vi "UDP Data Link - Driver Utilities - Launch Asynch UDP Loop.vi"(4 "In4Ver":u16, 5 "Rx Initial Values":dbl[](array[numeric]), 6 "SourceNodeName":string, 7 "Status Notifier":refnum<notifier>, 8 "error in (no error)":errorcluster, 9 "Rx Data FIFO":refnum<k33>, 10 "Tx Data FIFO":refnum<k33>, 11 "Device Reference in":T1 format="%.0x") -> (0 "error out":errorcluster)   [LabVIEW 2012, in "UDP Data Link Engine.lvlib"]
doc: "This VI launches the Asynchronous UDP Loop VI in a parallel data space. Before running the asynch VI, it initializes the input data on that VI with the Rx and Tx Data FIFO references, SourceNodeName, In4Ver, UDP Port, IP of Local NIC, and IP of Simulation Machine."
uses:
  UDP Data Link Engine.lvlib
  <vilib>/NI Veristand/Custom Device API/Custom Device Item Ref.ctl
  Shared/UDP Data Link Global.vi
  <vilib>/NI Veristand/Custom Device API/Get Item Property (U16).vi
  <vilib>/NI Veristand/Custom Device API/Get Item Property (String).vi
  UDP Data Link - Driver Utilities - Asynch UDP Loop.vi
  <vilib>/NI Veristand/Custom Device API/Custom Device API.lvlib
  Shared/UDP Data Link Shared.lvlib
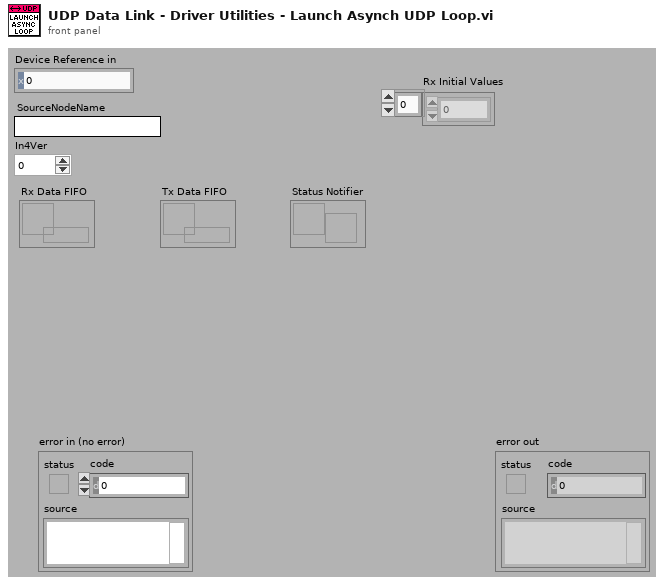
[diagram p1: front panel]
types:
  T1 = typedef "Custom Device API.lvlib/Custom Device Item Ref.ctl" = u64
  T2 = cluster{"Value":string, "Value":string, "Value":u16, "Rx Data FIFO":refnum<k33>, "Tx Data FIFO":refnum<k33>, "SourceNodeName":string, "In4Ver":u16, "Status Notifier":refnum<notifier>, "Rx Initial Values":dbl[]}
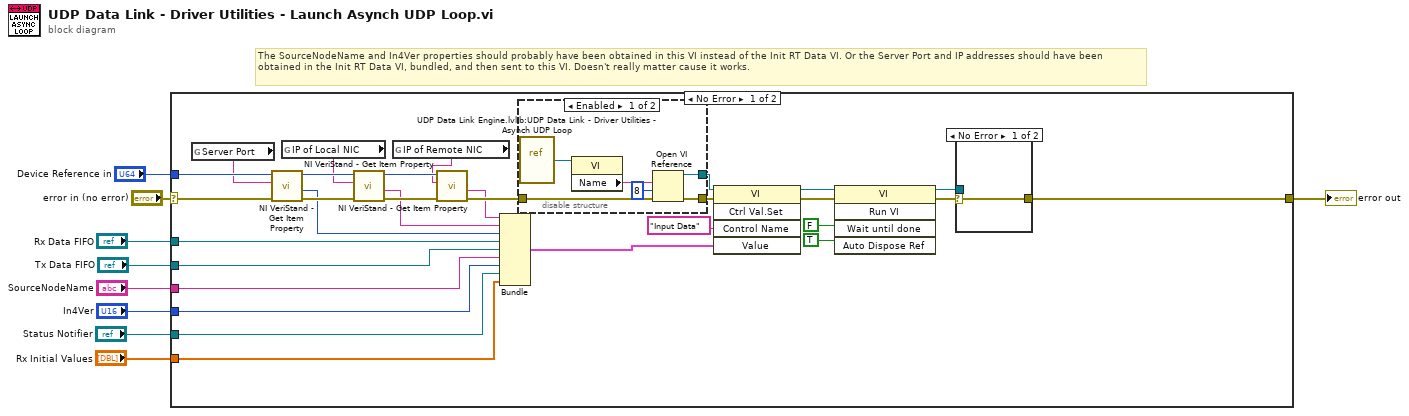
[diagram p0: block diagram]
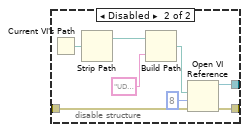
[diagram p2: hidden frame]
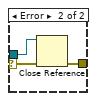
[diagram p3: hidden frame]
diagram:
  # "The SourceNodeName and In4Ver properties should probably have been obtained in this VI instead of the Init RT Data VI. Or the Server Port and IP addresses should have been obtained in the Init RT Data VI, bundled, and then sent to this VI. Doesn't really matter cause it works."
  n1 = case shown="No Error" "error in (no error)" {
    selector: "error in (no error)" -> [w20 w58]
    tunnel: [w29 w58] -> w8
    tunnel: "Rx Data FIFO" -> [w28 _]
    tunnel: "Tx Data FIFO" -> [w27 _]
    tunnel: "Device Reference in" -> [w21 _]
    tunnel: "In4Ver" -> [w16 _]
    tunnel: "SourceNodeName" -> [w15 _]
    tunnel: "Status Notifier" -> [w13 _]
    tunnel: "Rx Initial Values" -> [w12 _]
    frame No Error {
      n2 = global read "UDP Data Link Global.vi" "Server Port"() -> (w14:string)
      n3 = call-poly <vilib>:"NI VeriStand - Get Item Property.vi"("error in (no error)"=w20, "Property Name"=w14, "Item Ref in"=w21) -> ("error out"=w19:errorcluster, "Value"=w17:u16, "Item Ref out"=w18:T1)  [unwired: 5 in, 1 out]
      n4 = global read "UDP Data Link Global.vi" "IP of Local NIC"() -> (w11:string)
      n5 = call-poly <vilib>:"NI VeriStand - Get Item Property.vi"("error in (no error)"=w19, "Property Name"=w11, "Item Ref in"=w18) -> ("error out"=w26:errorcluster, "Value"=w23:string, "Item Ref out"=w22:T1)  [unwired: 5 in, 1 out]
      n6 = global read "UDP Data Link Global.vi" "IP of Remote NIC"() -> (w10:string)
      n7 = call-poly <vilib>:"NI VeriStand - Get Item Property.vi"("error in (no error)"=w26, "Property Name"=w10, "Item Ref in"=w22) -> ("error out"=w25:errorcluster, "Value"=w24:string)  [unwired: 5 in, 2 out]
      n8 = Bundle("Value"=w24, "Value"=w23, "Value"=w17, "Rx Data FIFO"=w28, "Tx Data FIFO"=w27, "SourceNodeName"=w15, "In4Ver"=w16, "Status Notifier"=w13, "Rx Initial Values"=w12) -> (w35:T2)  [unwired: 1 out]
      n9 = disable-structure shown="Enabled" {
        disable-tunnel: [w45 w52] -> w39
        disable-tunnel: [w44 w51] -> w38
        disable-tunnel: w25 -> [w43 w50]
        frame Enabled {
          n10 = vi-ref "UDP Data Link Engine.lvlib:UDP Data Link - Driver Utilities - Asynch UDP Loop.vi"() -> (w42:refnum<vi>)
          n11 = property class="VI"(reference=w42) -> ("Name"=w41:string)  [unwired: 1 in, 2 out]
          n12 = Open VI Reference(vi path=w41, options=8, error in (no error)=w43) -> (vi reference=w45:refnum<vi>, error out=w44:errorcluster)  [unwired: 3 out]
        }
        frame Disabled {
          n13 = Current VI's Path() -> (path=w49:path)
          n14 = Strip Path(path=w49) -> (stripped path=w48:path)  [unwired: 1 out]
          n15 = Build Path(base path=w48, name or relative path="UDP - Deterministic Communication - Test Utilities - Asynch FIFO Loop.vi") -> (appended path=w47:path)
          n16 = Open VI Reference(vi path=w47, options=8, error in (no error)=w50) -> (vi reference=w52:refnum<vi>, error out=w51:errorcluster)  [unwired: 1 in, 2 out]
        }
      }
      n17 = invoke class="VI" method="Ctrl Val.Set"(reference=w39, error in=w38, "Control Name"="Input Data", "Value"=w35) -> (reference out=w36:refnum<vi>, error out=w37:errorcluster)  [unwired: 1 in, 3 out]
      n18 = invoke class="VI" method="Run VI"(reference=w36, error in=w37, "Wait until done"=FALSE ("Wait Until Done"), "Auto Dispose Ref"=TRUE ("Auto Dispose Reference")) -> (reference out=w34:refnum<vi>, error out=w33:errorcluster)  [unwired: 1 in, 3 out]
      n19 = case shown="No Error" w33 {
        selector: w33 -> [w54 w57]
        tunnel: w34 -> [_ w56]
        tunnel: [w54 w55] -> w29
        frame No Error {
        }
        frame Error {
          n20 = Close Reference(reference=w56, error in (no error)=w57) -> (error out=w55:errorcluster)
        }
      }
    }
    frame Error {
    }
  }
  "error out" <- w8
